vi "Read Df.vi"(8 "error in (no error)":errorcluster, 11 "Send New Chirp MSG in":refnum<class "Send New Chirp MSG.lvclass">) -> (0 "error out":errorcluster, 2 "Df":i16, 3 "Send New Chirp MSG out":refnum<class "Send New Chirp MSG.lvclass">)   [LabVIEW 2014, in "ePAS Library.lvlib" / "Send New Chirp MSG.lvclass"]
uses:
  Send New Chirp MSG.lvclass
  Send New Chirp MSG.lvclass/Send New Chirp MSG.ctl
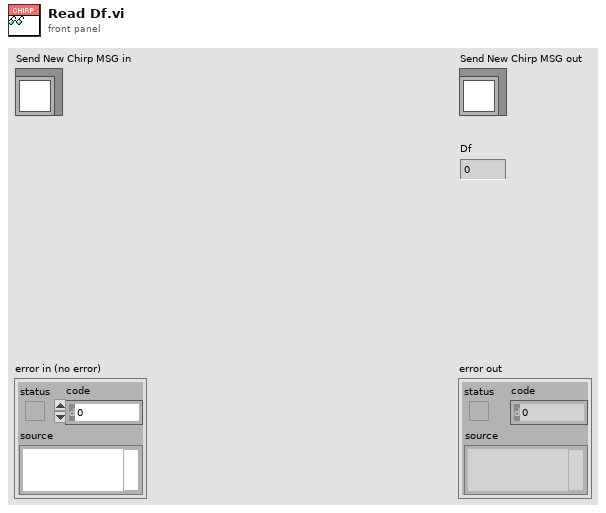
[diagram p1: front panel]
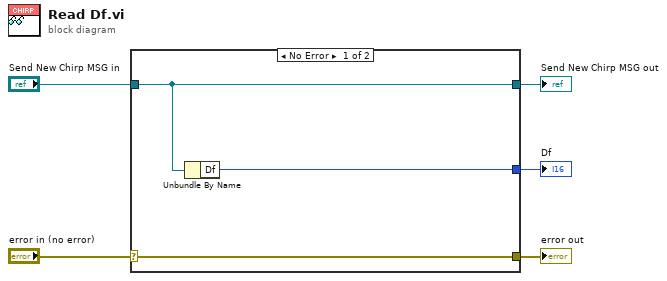
[diagram p0: block diagram]
diagram:
  n1 = case shown="No Error" "error in (no error)" {
    selector: "error in (no error)" -> [w8 w9]
    tunnel: [w8 w9] -> w4
    tunnel: [w7 w10] -> w2
    tunnel: "Send New Chirp MSG in" -> [w7 w10]
    tunnel: [w6 _] -> w1
    frame No Error {
      n2 = Unbundle By Name(w7) -> ("Df"=w6:i16)
    }
    frame Error {
    }
  }
  "error out" <- w4
  "Send New Chirp MSG out" <- w2
  "Df" <- w1
